vi "Initialize.vi"(8 "error in (no error)":errorcluster, 11 "WT1600.lvlib:WT1600.lvclass":refnum<class "WT1600.lvclass">) -> (0 "error out (no error)":errorcluster, 3 "WT1600.lvlib:WT1600.lvclass":refnum<class "WT1600.lvclass">)   [LabVIEW 2012, in "Universal Power Meter.lvlib" / "WT1600.lvlib" / "WT1600.lvclass"]
uses:
  WT1600.lvclass
  WT1600.lvclass/WT1600.ctl
  Global VI.vi
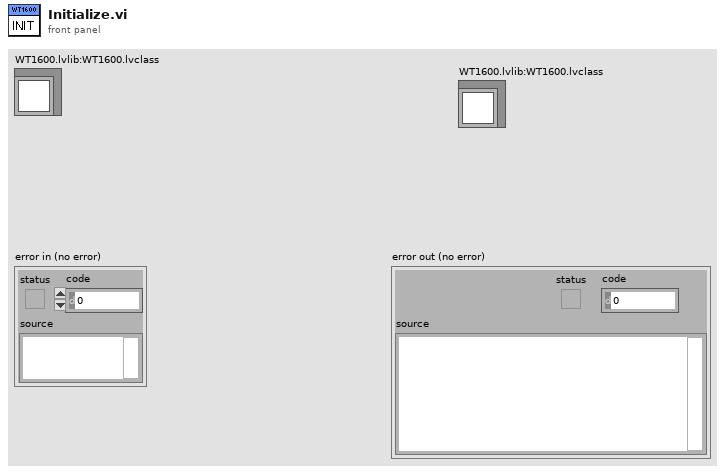
[diagram p1: front panel]
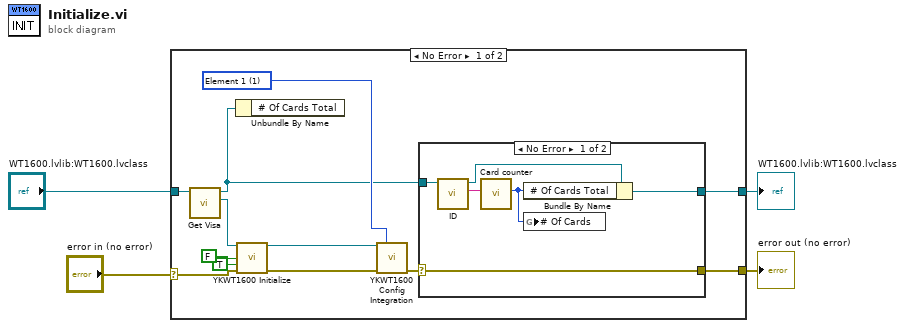
[diagram p0: block diagram]
diagram:
  n1 = case shown="No Error" "error in (no error)" {
    selector: "error in (no error)" -> [w15 w25]
    tunnel: "WT1600.lvlib:WT1600.lvclass" -> [w12 w26]
    tunnel: [w14 w26] -> w2
    tunnel: [w13 w25] -> w1
    frame No Error {
      w11 = u16 1 items=["All", "Element 1", "Element 2", "Element 3", "Element 4", "Element 5", "Element 6"] ("Element (0: All)")
      n2 = call "Get Visa.vi"("WT1600.lvlib:WT1600.lvclass"=w12) -> ("WT1600 Visa"=w8:refnum<visa-resource-name>, "WT1600.lvlib:WT1600.lvclass 2"=w9:refnum<class "WT1600.lvclass">)  [unwired: 9 in]
      n3 = Unbundle By Name(w9) -> ()  [unwired: 1 out]
      n4 = call <instrlib>:"YKWT1600 Initialize.vi"("VISA session (for class)"=w8, "ID Query (T: Check)"=FALSE, "Reset (T: Reset)"=TRUE, "error in (no error)"=w15) -> ("VISA session"=w6:refnum<visa-resource-name>, "error out"=w5:errorcluster)  [unwired: 10 in]
      n5 = call <instrlib>:"YKWT1600 Config Integration.vi"("VISA session"=w6, "Element (0: All)"=w11, "error in (no error)"=w5) -> ("error out"=w10:errorcluster)  [unwired: 11 in, 1 out]
      n6 = case shown="No Error" w10 {
        selector: w10 -> [w21 w23]
        tunnel: w9 -> [w22 w24]
        tunnel: [w18 w24] -> w14
        tunnel: [w21 w23] -> w13
        frame No Error {
          n7 = call "ID.vi"("WT1600.lvlib:WT1600.lvclass"=w22) -> ("Full ID"=w20:string, "WT1600.lvlib:WT1600.lvclass 2"=w19:refnum<class "WT1600.lvclass">)  [unwired: 9 in]
          n8 = call "Card counter.vi"("ID"=w20) -> ("# of Cards"=w17:i32)  [unwired: 10 in]
          n9 = Bundle By Name(cluster=w19, "# Of Cards Total"=w17) -> (w18:refnum<class "WT1600.lvclass">)
          n10 = global write "Global VI.vi" "# Of Cards"(w17) -> ()
        }
        frame Error {
        }
      }
    }
    frame Error {
    }
  }
  "error out (no error)" <- w1
  "WT1600.lvlib:WT1600.lvclass" <- w2
